vi "FTW-Actor-BeginShutdownSequence.vi"(1 "Jobs Prior to Shutdown Sequence":string, 3 "FTW Actor Instance":refnum<class "FTW-ActorInstance.lvclass">) -> (0 "FTW Actor Instance out":refnum<class "FTW-ActorInstance.lvclass">)   [LabVIEW 2013, in "FTW-ActorInstance.lvclass"]
uses:
  FTW-ActorInstance.lvclass
  FTW-ActorInstance.lvclass/FTW-ActorInstance.ctl
  JobSequencer/FTW-JobSequencer.lvclass
panel:
  # "Inputs"
  # "Outputs"
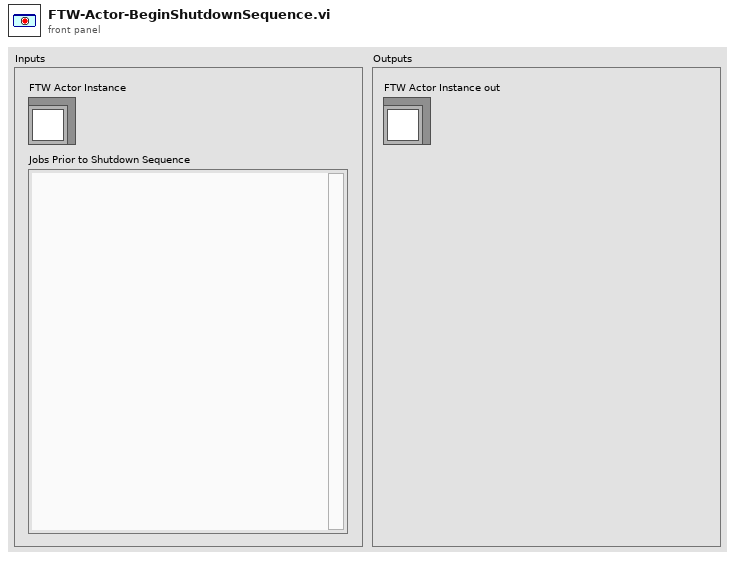
[diagram p1: front panel]
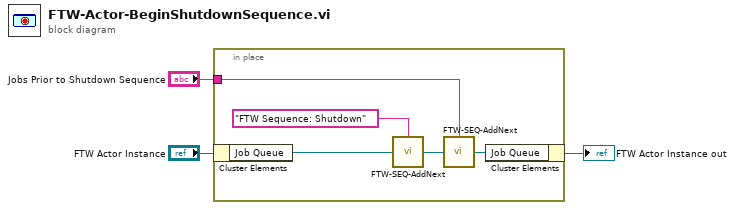
[diagram p0: block diagram]
diagram:
  n1 = in-place {
    in-place-border: "Jobs Prior to Shutdown Sequence" -> [w7]
    n2 = in-place-cluster #1("FTW Actor Instance") -> ("Job Queue"=w6:refnum<class "FTW-JobSequencer.lvclass">)
    n3 = call "FTW-SEQ-AddNext.vi"("Add Next in Sequence"="FTW Sequence: Shutdown", "FTW Job Sequencer"=w6) -> ("FTW Job Sequencer out"=w5:refnum<class "FTW-JobSequencer.lvclass">)  [unwired: 2 in]
    n4 = call "FTW-SEQ-AddNext.vi"("Add Next in Sequence"=w7, "FTW Job Sequencer"=w5) -> ("FTW Job Sequencer out"=w8:refnum<class "FTW-JobSequencer.lvclass">)  [unwired: 2 in]
    n5 = in-place-cluster #1("Job Queue"=w8) -> (→"FTW Actor Instance out":refnum<class "FTW-ActorInstance.lvclass">)
  }
